vi "niRFUtil RFHS Util Assert.vi"(11 "error constant":errorcluster, 13 "valid?":bool) -> (15 "error constant 3":errorcluster)   [LabVIEW 2015, in "niRFUtil.lvlib"]
uses:
  niRFUtil.lvlib
  Channelizer/Includes/niRFUtil RFHS Channelizer ChannelizerErrors.ctl
panel:
  # "Use this VI like you use assert(bool) in C.\nIf you just call it, it will generate an error\nor even trigger a breakpoint. \n\nYou can use it to have one single place\nwhere you enable this type of interruption, \nso we can effectivly disable the breakpoint\non releasing."
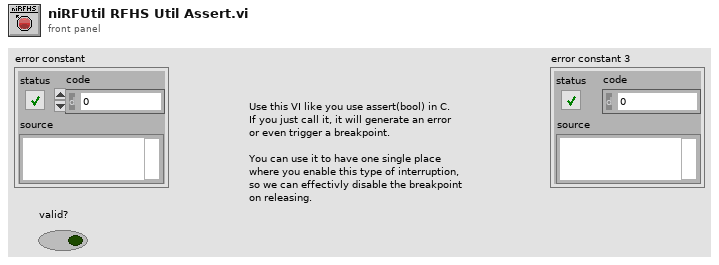
[diagram p1: front panel]
types:
  T1 = typedef "niRFUtil.lvlib/niRFUtil RFHS Channelizer ChannelizerErrors.ctl" = enum32{"No Error", "Invalid Channel", "Internal Error", "Invalid Channel fs", "Invalid Phase Shift", "Invalid fs", "Invalid Number Of Channles", "Invalid FFT Channel fs", "Invalid Resampler Channel fs", "Not a 15kHz Multiple", "Invalid Channel fc", "Invalid passBW/stopBW", "Coerced Rejection", "Requires Internal Buffer", "Duplicated Destination Channel Name", "Configuration Format Error", "Illegal Execution state", "DLL not found", "DLL loading failure", "AVX instruction failure"}
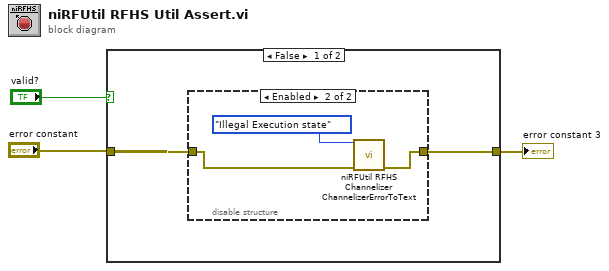
[diagram p0: block diagram]
diagram:
  n1 = case shown="False" "valid?" {
    tunnel: "error constant" -> [w5 w10]
    tunnel: [w4 w10] -> w1
    frame False {
      n2 = disable-structure shown="Enabled" {
        disable-tunnel: w5 -> [w6 w9]
        disable-tunnel: [w6 w8] -> w4
        frame Disabled {
        }
        frame Enabled {
          n3 = call "niRFUtil RFHS Channelizer ChannelizerErrorToText.vi"("Error List"=niRFUtil_RFHS_Channelizer_ChannelizerErrors."Illegal Execution state", "error in (no error)"=w9) -> ("error out"=w8:errorcluster)  [unwired: 13 in]
        }
      }
    }
    frame True {
    }
  }
  "error constant 3" <- w1
